vi "Actor Simple Sending.vi"(7 "System Actor In":refnum<class "System Actor.lvclass">, 8 "error in (no error)":errorcluster, 10 "Sending ID":i64, 11 "Self Addressed Task in":refnum<class "Self Addressed Task.lvclass">) -> (0 "error out":errorcluster, 3 "Self Addressed Task out":refnum<class "Self Addressed Task.lvclass">, 5 "System Actor Out":refnum<class "System Actor.lvclass">)   [LabVIEW 2024, in "Self Addressed Task.lvclass"]
uses:
  Self Addressed Task.lvclass
  Self Addressed Task.lvclass/Self Addressed Task.ctl
  Message/Message.lvclass
  Message/Type Def/CMD Type.ctl
  Message/Type Def/General CMD.ctl
  C:/Users/iio/Desktop/Bussiness/Tricorn Re/Madelbrot 4.0/General Library/Ancestor Class/Task/Task Ancestor/Task Ancestor.lvclass
  C:/Users/iio/Desktop/Bussiness/Tricorn Re/Madelbrot 4.0/General Library/Ancestor Class/Task/Self Addressed Task/Self Addressed Task.lvclass
  Actor/System Actor/System Actor.lvclass
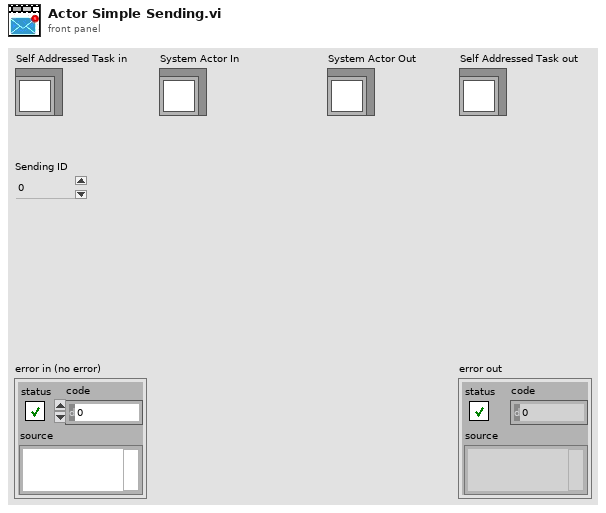
[diagram p1: front panel]
types:
  T1 = typedef "General CMD.ctl" = enum16{"None", "Stop", "Abort", "Running Task", "Running Batch Tasks", "Task Self Running", "Emergency Stop", "Subscribe", "UnSubscribe", "Pause", "Receive Parameters", "Active", "Resume"}
  T2 = typedef "CMD Type.ctl" = enum16{"None", "General CMD", "1st CMD", "2nd CMD", "3rd CMD", "4th CMD", "5th CMD", "6th CMD", "7th CMD"}
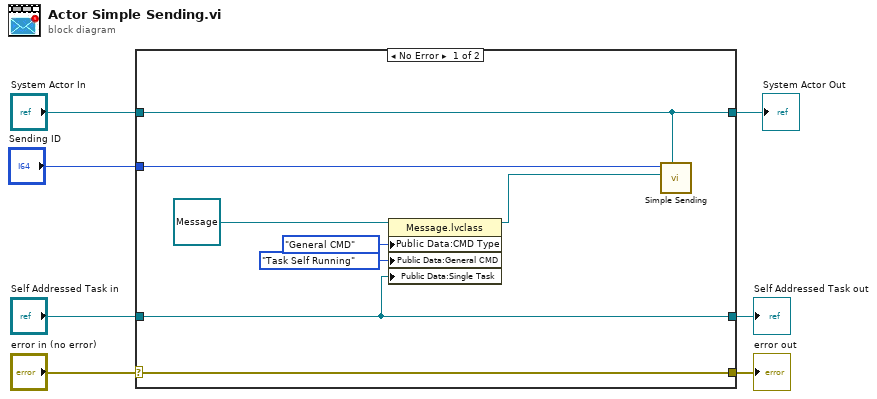
[diagram p0: block diagram]
diagram:
  n1 = case shown="No Error" "error in (no error)" {
    selector: "error in (no error)" -> [w15 w17]
    tunnel: [w15 w17] -> w6
    tunnel: [w11 w18] -> w4
    tunnel: "Self Addressed Task in" -> [w11 w18]
    tunnel: "System Actor In" -> [w14 w16]
    tunnel: [w14 w16] -> w2
    tunnel: "Sending ID" -> [w13 _]
    frame No Error {
      n2 = property class="Message.lvclass"(reference=refnum<class "Message.lvclass"> refnum ("Message.lvclass"), "Public Data:CMD Type"=CMD_Type."General CMD" ("CMD Type"), "Public Data:General CMD"=General_CMD."Task Self Running" ("General CMD"), "Public Data:Single Task"=w11) -> (reference out=w8:refnum<class "Message.lvclass">)  [unwired: 1 in, 1 out]
      n3 = call "Simple Sending.vi"("System Actor In"=w14, "Message In"=w8, "ID In"=w13) -> ()  [unwired: 9 in]
    }
    frame Error {
    }
  }
  "error out" <- w6
  "Self Addressed Task out" <- w4
  "System Actor Out" <- w2
